vi "_Read (No Objects) - Wavelength meter.vi"(8 "error in (no error)":errorcluster, 11 "Cluster In":T3={"Exp Range Min"=0, "Exp Range Max"=0, "exposure mode"=enum."manual", "operation (meas. mode)"=enum."Measurement mode", "Exposure (ms)"=0, "Quiet Errors?"=FALSE, "Error Status"={"status"=FALSE, "code"=0, "source"=""}}) -> (0 "error out":errorcluster, 2 "4 Data Points":dbl[](array[numeric]), 3 "Cluster Out":T3={"Exp Range Min"=0, "Exp Range Max"=0, "exposure mode"=enum."manual", "operation (meas. mode)"=enum."Measurement mode", "Exposure (ms)"=0, "Quiet Errors?"=FALSE, "Error Status"={"status"=FALSE, "code"=0, "source"=""}})   [LabVIEW 2012]
uses:
  HighFinesse WS5/Variable Typedefs.llb/Exposure Mode.ctl
  HighFinesse WS5/Control typedefs.llb/Measurement Mode.ctl
  HighFinesse WS5/HighFinesse WS5.lvlib
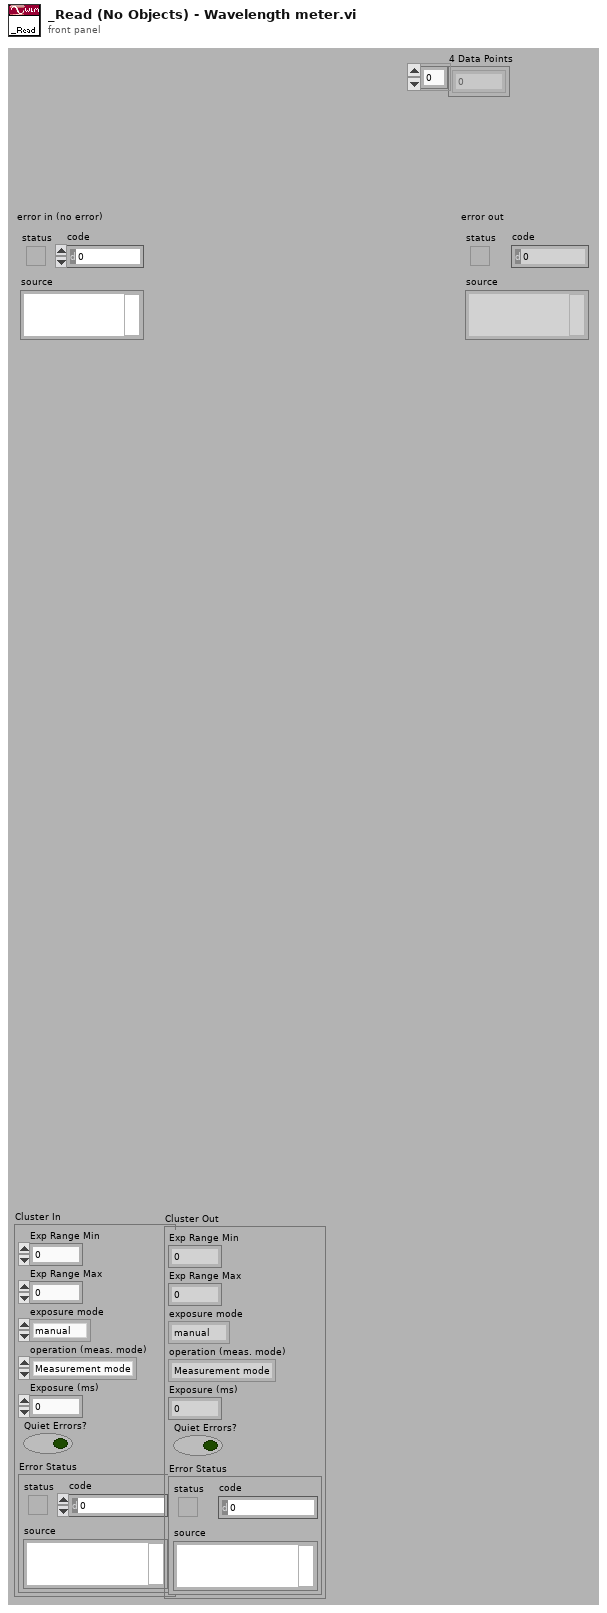
[diagram p1: front panel]
types:
  T1 = typedef "HighFinesse WS5.lvlib/Exposure Mode.ctl" = enum16{"manual", "automatic"}
  T2 = typedef "HighFinesse WS5.lvlib/Measurement Mode.ctl" = enum16{"Measurement off", "Adjustment mode", "Measurement mode"}
  T3 = cluster{"Exp Range Min":u32, "Exp Range Max":u32, "exposure mode":T1, "operation (meas. mode)":T2, "Exposure (ms)":u16, "Quiet Errors?":bool, "Error Status":errorcluster}
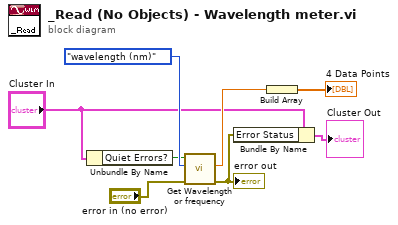
[diagram p0: block diagram]
diagram:
  n1 = Unbundle By Name("Cluster In") -> ("Quiet Errors?"=w5:bool)
  n2 = call "Get Wavelength or frequency.vi"("error in (no error)"="error in (no error)", "mode (wavelength)"=enum16{"wavelength (nm)", "frequency (THz)"}."wavelength (nm)", "Quiet Errors?"=w5) -> ("error out"=w4:errorcluster, "result"=w7:dbl)  [unwired: 1 in, 6 out]
  "error out" <- w4
  n3 = Bundle By Name(cluster="Cluster In", "Error Status"=w4) -> (→"Cluster Out":T3)
  n4 = Build Array(w7) -> (→"4 Data Points":dbl[])
